vi "Acquisition Message Loop.vi"(8 "error in (no error)":errorcluster, 11 "Message Queues":T1) -> (0 "error out":errorcluster)   [LabVIEW 2025, in "Acquisition.lvlib"]
doc: "Message loop for handling messages pertaining to the acquisition of data from the hardware."
uses:
  Acquisition.lvlib
  support/Message Queue/All Message Queues.ctl
  support/Message Queue/Message Cluster.ctl
  Acquistion_Configuration.ctl
  Signal Type.ctl
  Acquisition State.ctl
  support/Message Queue/Enqueue Message (Single).vi
  <vilib>/Utility/error.llb/Error Cluster From Error Code.vi
  <vilib>/ErrorRing/Error Ring.xnode
  support/Message Queue/Message Queue.lvlib
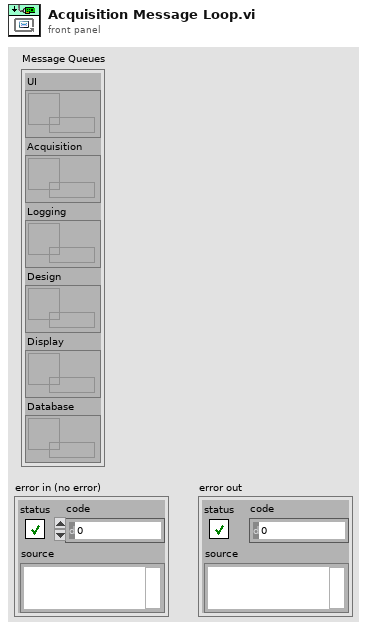
[diagram p1: front panel]
types:
  T1 = typedef "Message Queue.lvlib/All Message Queues.ctl" = cluster{"UI":refnum<queue>, "Acquisition":refnum<queue>, "Logging":refnum<queue>, "Design":refnum<queue>, "Display":refnum<queue>, "Database":refnum<queue>}
  T2 = typedef "Acquisition.lvlib/Acquistion_Configuration.ctl" = cluster{"HW Refnum":string, "Signal Type":T3, "Flow Rates":dbl[]}
  T3 = typedef "Acquisition.lvlib/Signal Type.ctl" = enum16{"Sine Wave", "Square with Noise"}
  T4 = typedef "Acquisition.lvlib/Acquisition State.ctl" = enum16{"Idle", "Acquiring"}
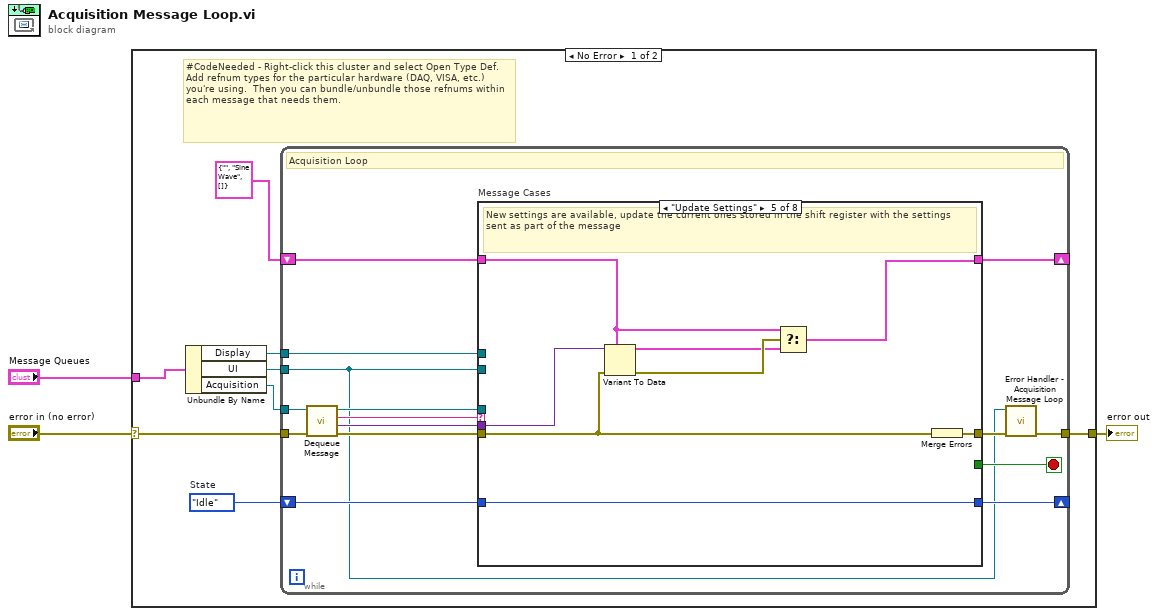
[diagram p0: block diagram]
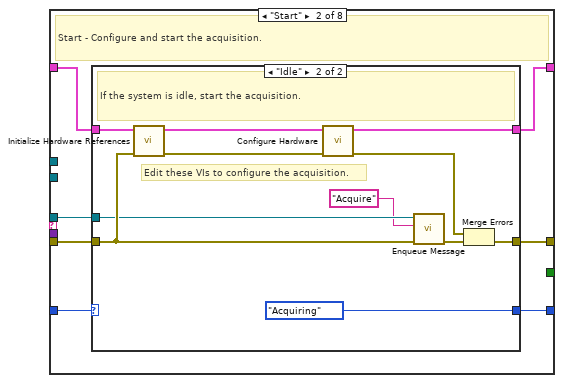
[diagram p3: hidden frame]
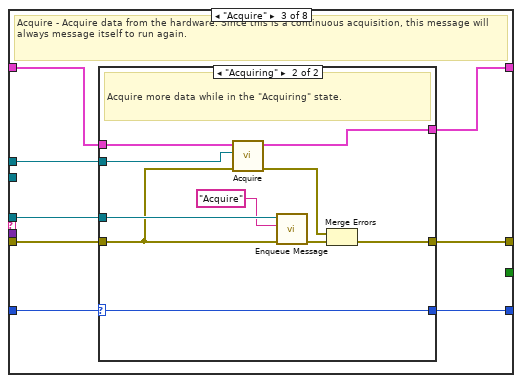
[diagram p5: hidden frame]
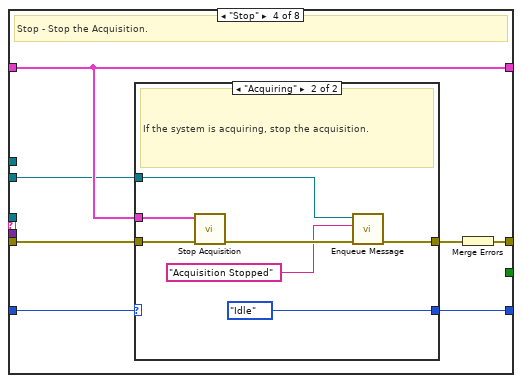
[diagram p7: hidden frame]
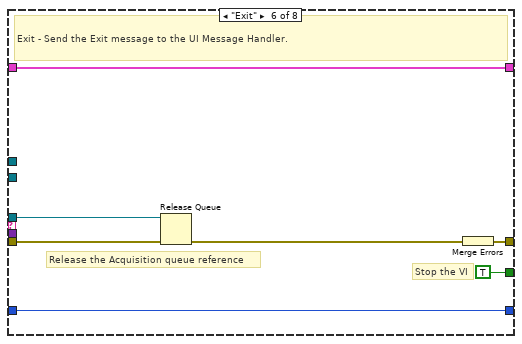
[diagram p9: hidden frame]
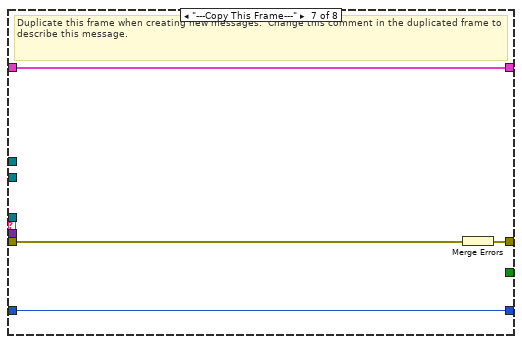
[diagram p10: hidden frame]
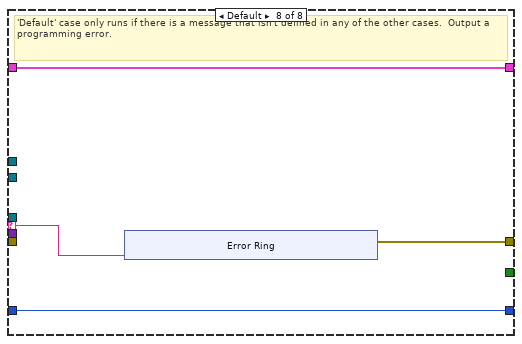
[diagram p11: hidden frame]
diagram:
  n1 = case shown="No Error" "error in (no error)" {
    selector: "error in (no error)" -> [w7 w118]
    tunnel: "Message Queues" -> [w11 _]
    tunnel: [w9 w118] -> w2
    frame No Error {
      w5 = Acquisition_State."Idle"  # State
      # "#CodeNeeded - Right-click this cluster and select Open Type Def.  Add refnum types for the particular hardware (DAQ, VISA, etc.) you're using.  Then you can bundle/unbundle those refnums within each message that needs them."
      n2 = Unbundle By Name(w11) -> ("Display"=w4:refnum<queue>, "UI"=w6:refnum<queue>, "Acquisition"=w10:refnum<queue>)
      n3 = while {
        tunnel: w10 -> [w19]
        shift-right: [w25] -> _
        shift-left: T2 {"HW Refnum"="", "Signal Type"=enum."Sine Wave", "Flow Rates"=[]} ("Data Cluster") -> [w26]
        tunnel: w6 -> [w13]
        shift-right: [w17] -> _
        shift-left: w5 -> [w18]
        tunnel: w7 -> [w23]
        tunnel: [w16] -> w9
        tunnel: w4 -> [w12]
        stop <- w24 stop-if-true
        # "Acquisition Loop"
        n4 = call "Dequeue Message.vi"("error in (no error)"=w23, "Message Queue"=w19) -> ("error out"=w22:errorcluster, "Message Data"=w20:variant, "Message"=w21:string, "dup Message Queue"=w14:refnum<queue>)  [unwired: 6 in]
        n5 = case "Message Cases" shown="\"Update Settings\"" w21 {
          selector: w21 -> [_ _ _ _ _ _ _ w107]
          tunnel: w14 -> [_ w33 w57 _ _ w97 _ _]
          tunnel: w22 -> [w29 w34 w56 w77 w89 w99 w106 _]
          tunnel: [w29 w36 w58 w78 w95 w101 w104 w108] -> w15
          tunnel: w26 -> [w28 w35 w54 w75 w91 w100 w105 w110]
          tunnel: [w28 w32 w55 w75 w90 w100 w105 w110] -> w25
          tunnel: [_ _ _ _ _ TRUE _ _] -> w24
          tunnel: w20 -> [_ _ _ _ w94 _ _ _]
          tunnel: w13 -> [_ _ _ w72 _ _ _ _]
          tunnel: w18 -> [w27 w30 w52 w74 w88 w96 w103 w109]
          tunnel: [w27 w31 w53 w73 w88 w96 w103 w109] -> w17
          tunnel: w12 -> [_ _ w51 _ _ _ _ _]
          frame "Initialize" {
            # "Initialize  - Initialize is currently a no-op.  The hardware initialization takes place in the 'Start' message."
          }
          frame "Start" {
            # "Start - Configure and start the acquisition."
            n6 = case shown="\"Idle\"" w30 {
              selector: w30 -> [w37 _]
              tunnel: [w38 w50] -> w36
              tunnel: w35 -> [w39 w49]
              tunnel: w34 -> [w38 w48]
              tunnel: w33 -> [_ w46]
              tunnel: [w39 w42] -> w32
              tunnel: [w37 Acquisition_State."Acquiring" ("Acquisition State")] -> w31
              frame "Acquiring" {
                # "The system is already acquiring. Ignore the \"Start\" message."
              }
              frame "Idle" {
                # "Edit these VIs to configure the acquisition."
                # "If the system is idle, start the acquisition."
                n7 = call "Initialize Hardware References.vi"("error in (no error)"=w48, "Hardware Resources in"=w49) -> ("error out"=w45:errorcluster, "Hardware Resources out"=w43:T2)  [unwired: 8 in]
                n8 = call "Configure Hardware.vi"("error in (no error)"=w45, "Hardware Resources in"=w43) -> ("error out"=w44:errorcluster, "Hardware Resources out"=w42:T2)  [unwired: 8 in]
                n9 = call-poly "Enqueue Message.vi"("error in (no error)"=w48, "Message"="Acquire", "Message Queue"=w46) -> ("error out"=w47:errorcluster)  [unwired: 7 in, 1 out]
                n10 = Merge Errors(w44, w47) -> (w50:errorcluster)
              }
            }
          }
          frame "Acquire" {
            # "Acquire - Acquire data from the hardware. Since this is a continuous acquisition, this message will always message itself to run again."
            n11 = case shown="\"Acquiring\"" w52 {
              selector: w52 -> [w59 w65]
              tunnel: [w60 w71] -> w58
              tunnel: w57 -> [_ w69]
              tunnel: w56 -> [w60 w64]
              tunnel: [w61 w67] -> w55
              tunnel: w54 -> [w61 w63]
              tunnel: [w59 w65] -> w53
              tunnel: w51 -> [_ w62]
              frame "Idle" {
                # "Ignore \"Acquire\" messages when the acquisition is idle."
              }
              frame "Acquiring" {
                # "Acquire more data while in the \"Acquiring\" state."
                n12 = call "Acquire.vi"("error in (no error)"=w64, "Display"=w62, "Hardware Resources in"=w63) -> ("error out"=w68:errorcluster, "Hardware Resources out"=w67:T2)  [unwired: 7 in]
                n13 = call-poly "Enqueue Message.vi"("error in (no error)"=w64, "Message"="Acquire", "Message Queue"=w69) -> ("error out"=w70:errorcluster)  [unwired: 7 in, 1 out]
                n14 = Merge Errors(w68, w70) -> (w71:errorcluster)
              }
            }
          }
          frame "Stop" {
            # "Stop - Stop the Acquisition."
            n15 = case shown="\"Acquiring\"" w74 {
              selector: w74 -> [w79 _]
              tunnel: w77 -> [w80 w87]
              tunnel: [w80 w83] -> w76
              tunnel: w75 -> [_ w85]
              tunnel: [w79 Acquisition_State."Idle" ("State")] -> w73
              tunnel: w72 -> [_ w82]
              frame "Idle" {
                # "The system is already idle. Ignore the \"Stop\" message."
              }
              frame "Acquiring" {
                # "If the system is acquiring, stop the acquisition."
                n16 = call "Stop Acquisition.vi"("error in (no error)"=w87, "Hardware Resources in"=w85) -> ("error out"=w86:errorcluster)  [unwired: 9 in]
                n17 = call-poly "Enqueue Message.vi"("error in (no error)"=w86, "Message"="Acquisition Stopped", "Message Queue"=w82) -> ("error out"=w83:errorcluster)  [unwired: 7 in, 1 out]
              }
            }
            n18 = Merge Errors(w76) -> (w78:errorcluster)
          }
          frame "Update Settings" {
            # "New settings are available, update the current ones stored in the shift register with the settings sent as part of the message"
            n19 = Variant To Data(error in=w89, type=w91, Variant=w94) -> (data=w92:T2, error out=w93:errorcluster)
            n20 = Select(t=w91, s=w93, f=w92) -> (s? t:f=w90:T2)
            n21 = Merge Errors(w89) -> (w95:errorcluster)
          }
          frame "Exit" {
            # "Release the Acquisition queue reference"
            # "Stop the VI"
            # "Exit - Send the Exit message to the UI Message Handler."
            n22 = Release Queue(queue=w97, error in (no error)=w99) -> (error out=w98:errorcluster)  [unwired: 1 in, 2 out]
            n23 = Merge Errors(w98) -> (w101:errorcluster)
          }
          frame "---Copy This Frame---" {
            # "Duplicate this frame when creating new messages.  Change this comment in the duplicated frame to describe this message."
            n24 = Merge Errors(w106) -> (w104:errorcluster)
          }
          frame Default {
            # "'Default' case only runs if there is a message that isn't defined in any of the other cases.  Output a programming error."
            n25 = xnode "Error Ring"("parameter 0"=w107) -> ("error out"=w108:errorcluster)
          }
        }
        n26 = call "Error Handler - Acquisition Message Loop.vi"("error in (no error)"=w15, "Message Queue"=w13) -> ("dup error in"=w16:errorcluster)  [unwired: 8 in, 1 out]
      }
    }
    frame Error {
    }
  }
  "error out" <- w2
